vi "Day 11 Puzzle 2.vi"(11 "Path":path) -> ()   [LabVIEW 2021]
uses:
  2502efef-52cf-4e36-8a2b-24fad6cf7fcc.vi
  <vilib>/Utility/file.llb/Read Delimited Spreadsheet (string).vi
  <vilib>/Comparison/Less/Less Functor/Less Functor.lvclass
panel:
  in  "Numeric":i32=1
  out "Array 2":i64[](array[numeric])
  out "Array":T1(array[cluster])
  out "Monkey business":i64
  out "length":i32
  out "deleted portion":string[](array[string])
  out "array w/ subset deleted":string[](array[string])
  out "all rows":string[][](array[string])
  out "subarray":string[](array[string])
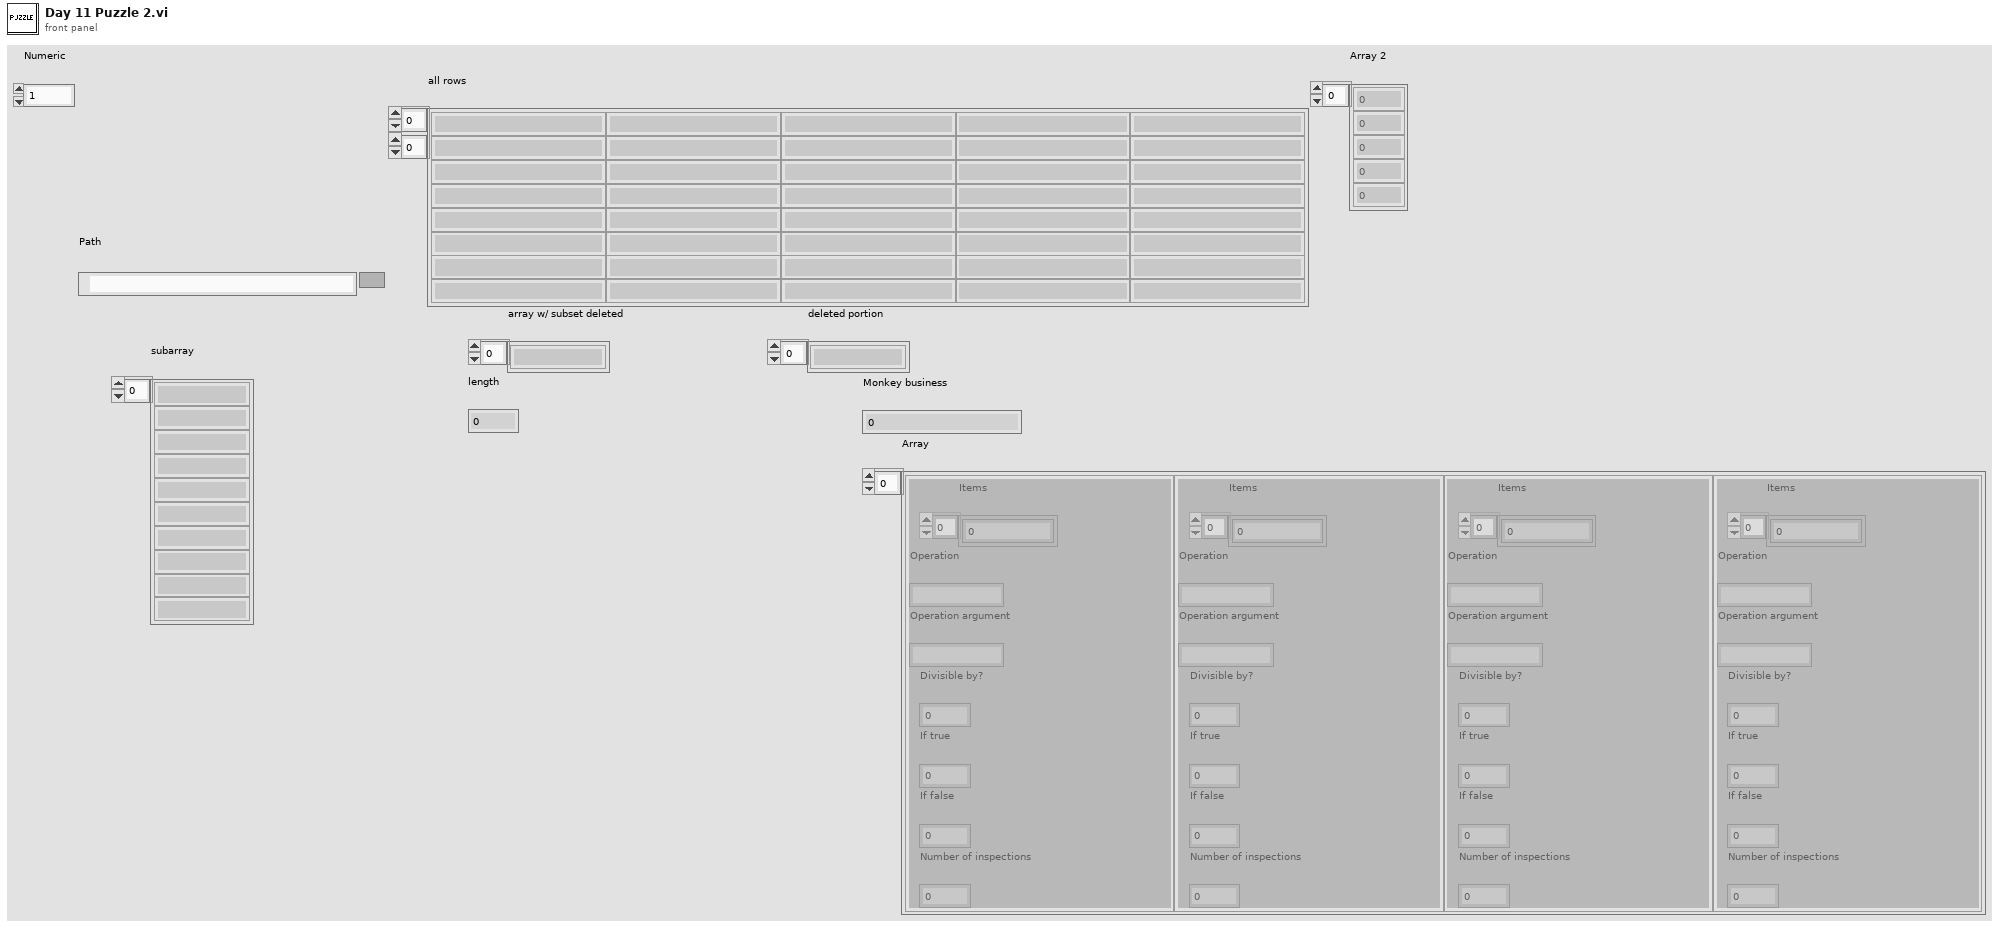
[diagram p1: front panel]
types:
  T1 = cluster{"Items":i32[], "Operation":string, "Operation argument":string, "Divisible by?":i32, "If true":i32, "If false":i32, "Number of inspections":i64}[]
  T2 = cluster{"Items":ext[], "Operation":string, "Operation argument":string, "Divisible by?":i32, "If true":i32, "If false":i32, "Number of inspections":i64}
  T3 = cluster{"Items":ext[], "Operation":string, "Operation argument":string, "Divisible by?":i32, "If true":i32, "If false":i32, "Number of inspections":i64}[]
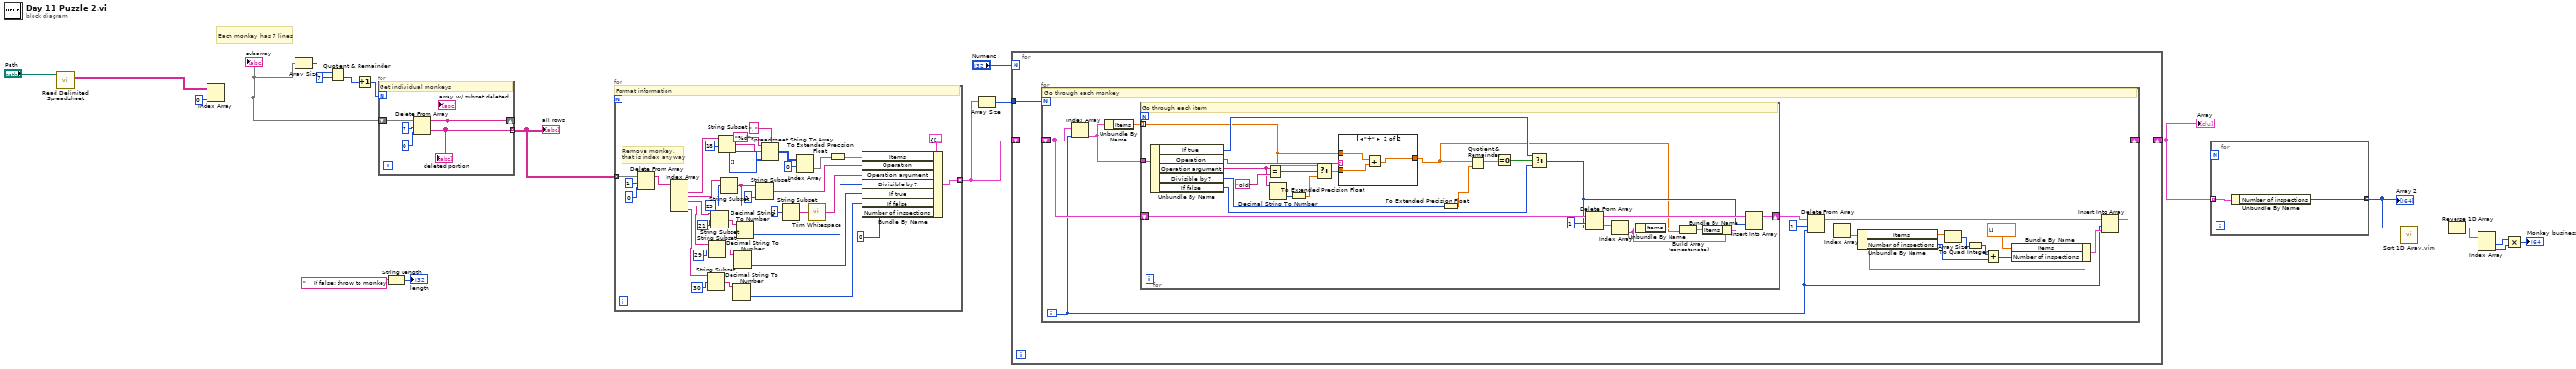
[diagram p0: block diagram]
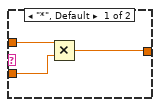
[diagram p2: hidden frame]
diagram:
  # "Each monkey has 7 lines"
  n1 = call-poly <vilib>:"Read Delimited Spreadsheet.vi"("file path (dialog if empty)"="Path") -> ("all rows"=w21:string[][])  [unwired: 9 in, 5 out]
  n2 = Index Array(array=w21, index (col)=0 ("disabled index (col)")) -> (element=w18:string[])  [unwired: 1 in]
  "subarray" <- w18
  n3 = Array Size(array=w18) -> (size(s)=w17:i32)
  n4 = Quotient & Remainder(x=w17, y=7) -> (floor(x/y)=w15:i32)  [unwired: 1 out]
  n5 = Increment(x=w15) -> (x+1=w14:i32)
  n6 = for {
    N: w14 -> [_]
    shift-right: [w23] -> _
    shift-left: w18 -> [w26]
    tunnel: [w22] -> w13 mode=indexing
    # "Get individual monkeys"
    n7 = Delete From Array(array=w26, length=7 ("index"), index=0 ("length")) -> (deleted portion=w22:string[], array with subset deleted=w23:string[])
    "array w/ subset deleted" <- w23
    "deleted portion" <- w22
  }
  "all rows" <- w13
  n8 = String Length(string="    If false: throw to monkey ") -> (length=→"length":i32)
  n9 = for {
    tunnel: w13 -> [w63] mode=indexing
    tunnel: [w30] -> w9 mode=indexing
    # "Remove monkey, \nthat is index anyway"
    # "Format information"
    n10 = Delete From Array(array=w63, length=1, index=0) -> (array with subset deleted=w60:string[])  [unwired: 1 out]
    n11 = Index Array(array=w60) -> (element #1=w59:string, element #2=w51:string, element #3=w42:string, element #4=w37:string, element #5=w34:string)  [unwired: 5 in]
    n12 = String Subset(string=w34, offset (0)=30) -> (substring=w35:string)  [unwired: 1 in]
    n13 = String Subset(string=w37, offset (0)=29) -> (substring=w38:string)  [unwired: 1 in]
    n14 = String Subset(string=w42, offset (0)=21) -> (substring=w41:string)  [unwired: 1 in]
    n15 = String Subset(string=w59, offset (0)=18) -> (substring=w55:string)  [unwired: 1 in]
    n16 = String Subset(string=w51, offset (0)=23) -> (substring=w47:string)  [unwired: 1 in]
    n17 = Decimal String To Number(string=w35) -> (number=w32:i32)  [unwired: 2 in, 1 out]
    n18 = Decimal String To Number(string=w38) -> (number=w33:i32)  [unwired: 2 in, 1 out]
    n19 = Decimal String To Number(string=w41) -> (number=w40:i32)  [unwired: 2 in, 1 out]
    n20 = String Subset(string=w47, length (rest)=1 ("length (rest)")) -> (substring=w48:string)  [unwired: 1 in]
    n21 = Spreadsheet String To Array(delimiter (Tab)=", ", format string="%d", spreadsheet string=w55, array type (2D Dbl)=i32[][] []) -> (array=w53:i32[][])
    n22 = String Subset(string=w47, offset (0)=1) -> (substring=w45:string)  [unwired: 1 in]
    n23 = Index Array(array=w53, index (row)=0) -> (element=w28:i32[])  [unwired: 1 in]
    n24 = call <vilib>:"Trim Whitespace.vi"("string"=w45) -> ("trimmed string"=w44:string)  [unwired: 1 in]
    n25 = To Extended Precision Float(1:w28) -> (0:w27:ext[])
    n26 = Bundle By Name(cluster=T2 {"Items"=[], "Operation"="", "Operation argument"="", "Divisible by?"=0, "If true"=0, "If false"=0, "Number of inspections"=0} ("output cluster"), "Items"=w27, "Operation"=w48, "Operation argument"=w44, "Divisible by?"=w40, "If true"=w33, "If false"=w32, "Number of inspections"=i64 0) -> (w30:T2)
  }
  n27 = Array Size(array=w9) -> (size(s)=w10:i32)
  n28 = for {
    N: "Numeric" -> [_]
    tunnel: w10 -> [w66]
    shift-right: [w64] -> w7
    shift-left: w9 -> [w65]
    n29 = for {
      N: w66 -> [_]
      shift-right: [w73] -> w64
      shift-left: w65 -> [w81]
      i -> [w74]
      # "Go through each monkey"
      n30 = Index Array(array=w81, index=w74) -> (element=w82:T2)
      n31 = Unbundle By Name(w82) -> ("Items"=w83:ext[])
      n32 = for {
        tunnel: w83 -> [w95] mode=indexing
        tunnel: w82 -> [w109]
        shift-right: [w89] -> w76
        shift-left: w81 -> [w99]
        # "Go through each item"
        n33 = Unbundle By Name(w109) -> ("If true"=w101:i32, "Operation"=w108:string, "Operation argument"=w105:string, "Divisible by?"=w87:i32, "If false"=w100:i32)
        n34 = Equal?(x=w105, y="old") -> (x = y?=w106:bool)
        n35 = Decimal String To Number(string=w105) -> (number=w85:i32)  [unwired: 2 in, 1 out]
        n36 = To Extended Precision Float(1:w85) -> (0:w84:ext)
        n37 = Select(t=w95, s=w106, f=w84) -> (s? t:f=w104:ext)
        n38 = case shown="\"+\"" w108 {
          tunnel: w104 -> [w111 w115]
          tunnel: w95 -> [w112 w114]
          tunnel: [w110 w113] -> w88
          frame "*", Default {
            n39 = Multiply(x=w112, y=w111) -> (x*y=w110:ext)
          }
          frame "+" {
            n40 = Add(x=w114, y=w115) -> (x+y=w113:ext)
          }
        }
        n41 = To Extended Precision Float(1:w87) -> (0:w86:ext)
        n42 = Quotient & Remainder(x=w88, y=w86) -> (x-y*floor(x/y)=w103:ext)  [unwired: 1 out]
        n43 = Equal To 0?(x=w103) -> (x = 0?=w102:bool)
        n44 = Select(t=w101, s=w102, f=w100) -> (s? t:f=w91:i32)
        n45 = Delete From Array(array=w99, length=1, index=w91) -> (deleted portion=w97:T3, array with subset deleted=w92:T3)
        n46 = Index Array(array=w97) -> (element=w94:T2)  [unwired: 1 in]
        n47 = Unbundle By Name(w94) -> ("Items"=w96:ext[])
        n48 = Build Array (concatenate)(w96, w88) -> (w93:ext[])
        n49 = Bundle By Name(cluster=w94, "Items"=w93) -> (w90:T2)
        n50 = Insert Into Array(array=w92, index=w91, new element=w90) -> (w89:T3)
      }
      n51 = Delete From Array(array=w76, length=1, index=w74) -> (deleted portion=w79:T3, array with subset deleted=w78:T3)
      n52 = Index Array(array=w79) -> (element=w72:T2)  [unwired: 1 in]
      n53 = Unbundle By Name(w72) -> ("Items"=w71:ext[], "Number of inspections"=w70:i64)
      n54 = Array Size(array=w71) -> (size(s)=w68:i32)
      n55 = To Quad Integer(1:w68) -> (0:w67:i64)
      n56 = Add(x=w67, y=w70) -> (x+y=w69:i64)
      n57 = Bundle By Name(cluster=w72, "Items"=ext[] [], "Number of inspections"=w69) -> (w77:T2)
      n58 = Insert Into Array(array=w78, index=w74, new element=w77) -> (w73:T3)
    }
  }
  "Array" <- w7
  n59 = for {
    tunnel: w7 -> [w117] mode=indexing
    tunnel: [w116] -> w6 mode=indexing
    n60 = Unbundle By Name(w117) -> ("Number of inspections"=w116:i64)
  }
  "Array 2" <- w6
  n61 = call "Sort 1D Array.vim"("unsorted array"=w6) -> ("sorted array"=w5:i64[])  [unwired: 10 in]
  n62 = Reverse 1D Array(array=w5) -> (reversed array=w4:i64[])
  n63 = Index Array(array=w4) -> (element #1=w3:i64, element #2=w2:i64)  [unwired: 2 in]
  n64 = Multiply(x=w3, y=w2) -> (x*y=→"Monkey business":i64)
